vi "Solver VI Type.vi"(11 "Feedback":string) -> (3 "Guess":string)   [LabVIEW 2024]
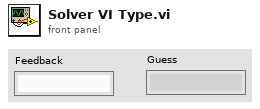
[diagram p1: front panel]
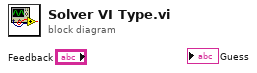
[diagram p0: block diagram]
diagram:
